vi "Read DIO from Parent.vi"(8 "error in":errorcluster, 11 "Data Value Reference in":refnum<data-value>) -> (0 "error out":errorcluster, 3 "DIO Lines":string[](array[string]))   [LabVIEW 2014, in "Bus.lvclass"]
uses:
  Bus.lvclass
  RIO Target/RIO Target.lvclass
  RIO Target Configuration/RIO Target Configuration.lvclass
  <vilib>/NI/Configuration Framework/serializable configuration/read metadata property.vi
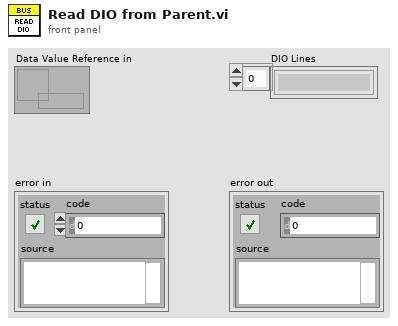
[diagram p1: front panel]
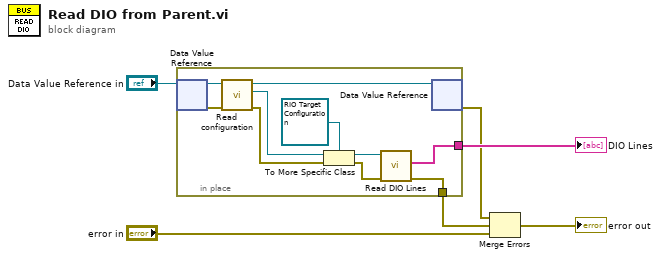
[diagram p0: block diagram]
diagram:
  n1 = in-place {
    in-place-border: [w12] -> w6
    in-place-border: [w7] -> w3
    n2 = in-place-dvr #1("Data Value Reference in") -> (w16:refnum<class "RIO Target.lvclass">, w10:errorcluster)
    n3 = call-dynamic "Read configuration.vi"("error in"=w10, "RIO Target in"=w16) -> ("error out"=w9:errorcluster, "configuration"=w15:refnum<class "NISE_CEF_serializable configuration.lvclass">, "RIO Target out"=w11:refnum<class "RIO Target.lvclass">)  [unwired: 7 in]
    n4 = To More Specific Class(target class=refnum<class "RIO Target Configuration.lvclass"> refnum ("RIO Target Configuration.lvclass"), reference=w15, error in=w9) -> (specific class reference=w13:refnum<class "RIO Target Configuration.lvclass">, error out=w8:errorcluster)
    n5 = call "Read DIO Lines.vi"("error in (no error)"=w8, "RIO Target Configuration in"=w13) -> ("error out"=w7:errorcluster, "DIO Lines"=w12:string[])  [unwired: 7 in, 1 out]
    n6 = in-place-dvr #1(w11) -> (w4:errorcluster)  [unwired: 1 out]
  }
  "DIO Lines" <- w6
  n7 = Merge Errors(w4, w3, "error in") -> (→"error out":errorcluster)
